vi "Disconnect.vi"(8 "error in":errorcluster, 11 "EF20 in":refnum<class "EF20.lvclass">) -> (0 "error out":errorcluster, 3 "EF20 out":refnum<class "EF20.lvclass">)   [LabVIEW 2018, in "EF20.lvlib" / "EF20.lvclass"]
uses:
  EF20.lvclass
  PPLs/Oven/Oven.lvlibp/Oven.lvclass
  PPLs/Oven/Oven.lvlibp/Custom Controls/Message Type.ctl
  PPLs/Oven/Oven.lvlibp
  C:/Projects/LabVIEW/PPLs/Oven/Oven.lvlibp/Oven.lvclass
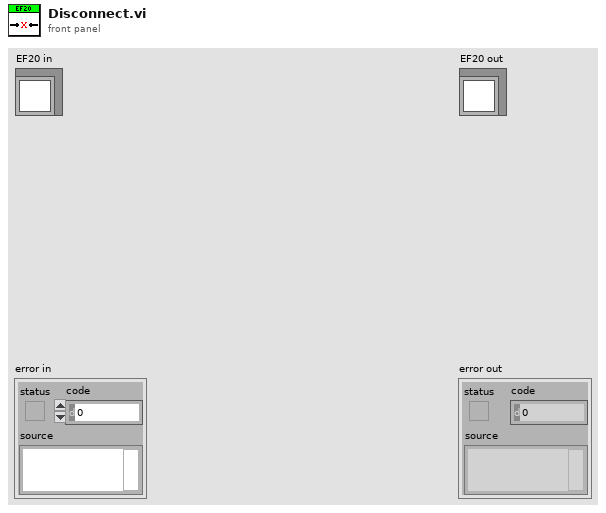
[diagram p1: front panel]
types:
  T1 = typedef "Oven.lvlibp/Message Type.ctl" = enum16{"Start", "Stop", "Set Temperature", "Get Temperature"}
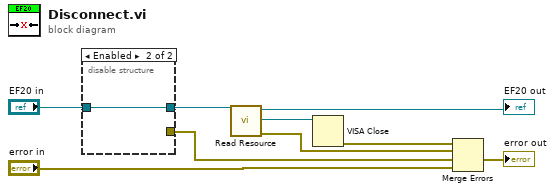
[diagram p0: block diagram]
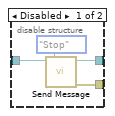
[diagram p2: hidden frame]
diagram:
  n1 = disable-structure shown="Enabled" {
    disable-tunnel: "EF20 in" -> [w13 w14]
    disable-tunnel: [w12 w14] -> w3
    disable-tunnel: [w11 _] -> w2
    frame Disabled {
      n2 = call-dynamic "Send Message.vi"("Message to Send"=Message_Type."Stop", "EF20 in"=w13) -> ("error out"=w11:errorcluster, "EF20 out"=w12:refnum<class "EF20.lvclass">)  [unwired: 8 in]
    }
    frame Enabled {
    }
  }
  n3 = call "Read Resource.vi"("Oven in"=w3) -> ("error out"=w6:errorcluster, "Resource"=w9:refnum<visa-resource-name>, "Oven out"=→"EF20 out":refnum<class "EF20.lvclass">)  [unwired: 8 in]
  n4 = VISA Close(VISA resource name=w9) -> (error out=w7:errorcluster)  [unwired: 1 in]
  n5 = Merge Errors(w7, w6, w2, "error in") -> (→"error out":errorcluster)
